vi "ExecuteMacrosRead.vi"(8 "error in (no error)":errorcluster, 11 "StepMotor in":refnum<class "StepMotor.lvclass">) -> (0 "error out":errorcluster, 2 "Значение":dbl, 3 "StepMotor out":refnum<class "StepMotor.lvclass">)   [LabVIEW 2010, in "StepMotor.lvclass"]
uses:
  StepMotor.lvclass
  StepMotor.lvclass/StepMotor.ctl
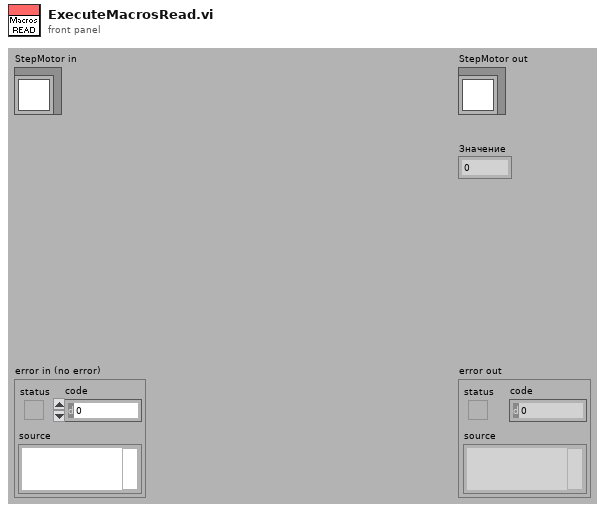
[diagram p1: front panel]
types:
  T1 = enum32{"cp1", "cp2", "cp3", "cp4", "cp5", "cp6", "cp7", "cp8", "cp9", "cp10", "cp11", "cp12", "vp1", "vp2", "vp16", "vp3", "vp4", "vp5", "vp6", "vp7", "vp8", "vp9", "vp10", "vp11", "vp12", "vp13", "vp14", "vp15", "vp17", "vp18", "vp19", "vp20", "vp21", "vp22", "vp23", "vp24", "vp25", "vp26", "pp1", "pp2", "pp3", "pp5", "pp6", "pp7", "pp8", "pp9", "pp10", "pp11", "ss1", "ss2", "ss3", "ss4", "ss5", "ss6", "ss7", "ss8", "ss9", "ss10", "ss11", "ss12", "ss13", "ss14", "ss15", "si1", "si2", "ss16", "ss17", "ss18", "ct1", "ct2", "ct3", "dd1", "dd6", "dd3", "dd9", "dd2", "dd4", "dd5", "dd21", "dd7", "dd8", "dd20", "dd10", "dd19", "dd12", "dd11", "dd13", "dd14", "dd15", "dd16", "dd17", "dd18", "dd22", "dd23", "dd24", "dd25", "dd26", "dd27", "dd28", "dd29", "dd30", "dd31", "dd32", "dd33", "dd34", "st1", "st2", "st3", "st4", "st5", "st6", "st7", "st8", "st9", "st10", "st11", "st12", "st13", "st14", "tp1", "tp3", "tp2", "tp5", "tp6", "ip0", "ip1", "ip2", "ip3", "ip4", "ip5", "ip6", "ip7", "ip8", "ip9", "ip10", "ip11", "ip12", "ip13", "ip14", "ip15", "ip16", "ip17", "ip18", "ip19", "ip20", "ep1", "ep2", "ep3", "ep4", "ep5", "ep6", "ep7", "up0", "up1", "up2", "up3", "up4", "up5", "up6", "up7", "up8", "up9", "up10", "up11", "up12", "up13", "up14", "up15", "up16", "up17", "up18", "up19", "up20", "up21", "up22", "up23", "up24", "io0", "io1", "io2", "io3", "io4", "io5", "io6", "io7", "io8", "io9", "io10", "io11", "io12", "io13", "io14", "pd1", "pd2", "pd3", "pd4", "pd5", "pd6", "pd7", "pd8", "pd9", "pd10", "pd11", "pd12", "pd13", "pd14", "pd15", "pd16", "pd17", "pd18", "pd19", " "}
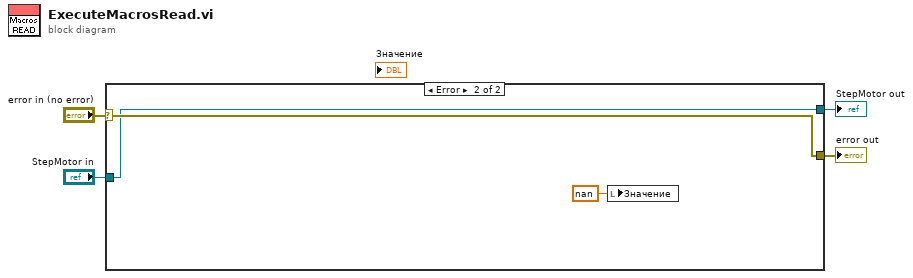
[diagram p0: block diagram]
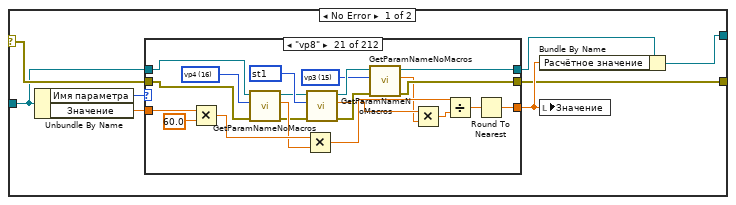
[diagram p2: hidden frame]
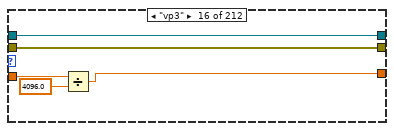
[diagram p18: hidden frame]
diagram:
  n1 = case shown="Error" "error in (no error)" {
    selector: "error in (no error)" -> [w10 w692]
    tunnel: [w9 w692] -> w3
    tunnel: [w12 w691] -> w1
    tunnel: "StepMotor in" -> [w8 w691]
    frame No Error {
      n2 = Unbundle By Name(w8) -> ("Имя параметра"=w5:T1, "Значение"=w6:dbl)
      n3 = case shown="\"vp8\"" w5 {
        tunnel: w6 -> [w15 w18 w21 w24 w27 w30 w33 w36 w39 w42 w45 w48 w51 w54 w57 w60 w63 w68 w71 w74 w83 w98 w101 w104 w107 w110 w124 w129 w132 w135 w138 w141 w144 w147 w150 w153 w156 w159 w162 w165 w168 w171 w174 w177 w180 w183 w186 w189 w192 w195 w198 w201 w204 w207 w210 w213 w216 w219 w222 w225 w228 w231 w234 w237 w240 w243 w246 w249 w252 w257 w260 w267 w270 w273 w276 w279 w282 w285 w288 w291 w294 w297 w301 w305 w308 w311 w314 w317 w320 w323 w326 w329 w332 w335 w338 w341 w344 w347 w350 w353 w356 w359 w362 w365 w368 w371 w374 w377 w380 w383 w386 w389 w392 w395 w398 w401 w404 w407 w410 w413 w416 w419 w422 w425 w428 w431 w434 w437 w440 w443 w446 w449 w452 w455 w458 w461 w464 w467 w470 w473 w476 w479 w482 w485 w488 w491 w494 w497 w500 w503 w506 w509 w512 w515 w518 w521 w524 w527 w530 w533 w536 w539 w542 w545 w548 w551 w554 w557 w560 w563 w566 w569 w572 w575 w578 w581 w584 w587 w590 w593 w596 w599 w602 w605 w608 w611 w614 w617 w620 w623 w626 w629 w632 w635 w638 w641 w644 w647 w650 w653 w656 w659 w662 w665 w668 w671 w674 w677 w680 w683 w686 w689]
        tunnel: [w15 w18 w21 w24 w27 w30 w33 w36 w39 w42 w45 w48 w51 w54 w57 w58 w63 w68 w71 w74 w84 w98 w101 w104 w107 w110 w111 w129 w132 w135 w138 w141 w144 w147 w150 w153 w156 w159 w162 w165 w168 w171 w174 w177 w180 w183 w186 w189 w192 w195 w198 w201 w204 w207 w210 w213 w216 w219 w222 w225 w228 w231 w234 w237 w240 w243 w246 w249 w252 w256 w260 w263 w270 w273 w276 w279 w282 w285 w288 w291 w294 w297 w300 w305 w308 w311 w314 w317 w320 w323 w326 w329 w332 w335 w338 w341 w344 w347 w350 w353 w356 w359 w362 w365 w368 w371 w374 w377 w380 w383 w386 w389 w392 w395 w398 w401 w404 w407 w410 w413 w416 w419 w422 w425 w428 w431 w434 w437 w440 w443 w446 w449 w452 w455 w458 w461 w464 w467 w470 w473 w476 w479 w482 w485 w488 w491 w494 w497 w500 w503 w506 w509 w512 w515 w518 w521 w524 w527 w530 w533 w536 w539 w542 w545 w548 w551 w554 w557 w560 w563 w566 w569 w572 w575 w578 w581 w584 w587 w590 w593 w596 w599 w602 w605 w608 w611 w614 w617 w620 w623 w626 w629 w632 w635 w638 w641 w644 w647 w650 w653 w656 w659 w662 w665 w668 w671 w674 w677 w680 w683 w686 w689] -> w11
        tunnel: w10 -> [w13 w16 w19 w22 w25 w28 w31 w34 w37 w40 w43 w46 w49 w52 w55 w61 w64 w66 w69 w72 w86 w96 w99 w102 w105 w108 w117 w127 w130 w133 w136 w139 w142 w145 w148 w151 w154 w157 w160 w163 w166 w169 w172 w175 w178 w181 w184 w187 w190 w193 w196 w199 w202 w205 w208 w211 w214 w217 w220 w223 w226 w229 w232 w235 w238 w241 w244 w247 w250 w253 w258 w261 w268 w271 w274 w277 w280 w283 w286 w289 w292 w295 w298 w303 w306 w309 w312 w315 w318 w321 w324 w327 w330 w333 w336 w339 w342 w345 w348 w351 w354 w357 w360 w363 w366 w369 w372 w375 w378 w381 w384 w387 w390 w393 w396 w399 w402 w405 w408 w411 w414 w417 w420 w423 w426 w429 w432 w435 w438 w441 w444 w447 w450 w453 w456 w459 w462 w465 w468 w471 w474 w477 w480 w483 w486 w489 w492 w495 w498 w501 w504 w507 w510 w513 w516 w519 w522 w525 w528 w531 w534 w537 w540 w543 w546 w549 w552 w555 w558 w561 w564 w567 w570 w573 w576 w579 w582 w585 w588 w591 w594 w597 w600 w603 w606 w609 w612 w615 w618 w621 w624 w627 w630 w633 w636 w639 w642 w645 w648 w651 w654 w657 w660 w663 w666 w669 w672 w675 w678 w681 w684 w687]
        tunnel: [w13 w16 w19 w22 w25 w28 w31 w34 w37 w40 w43 w46 w49 w52 w55 w61 w64 w66 w69 w72 w78 w96 w99 w102 w105 w108 w115 w127 w130 w133 w136 w139 w142 w145 w148 w151 w154 w157 w160 w163 w166 w169 w172 w175 w178 w181 w184 w187 w190 w193 w196 w199 w202 w205 w208 w211 w214 w217 w220 w223 w226 w229 w232 w235 w238 w241 w244 w247 w250 w253 w258 w261 w268 w271 w274 w277 w280 w283 w286 w289 w292 w295 w298 w303 w306 w309 w312 w315 w318 w321 w324 w327 w330 w333 w336 w339 w342 w345 w348 w351 w354 w357 w360 w363 w366 w369 w372 w375 w378 w381 w384 w387 w390 w393 w396 w399 w402 w405 w408 w411 w414 w417 w420 w423 w426 w429 w432 w435 w438 w441 w444 w447 w450 w453 w456 w459 w462 w465 w468 w471 w474 w477 w480 w483 w486 w489 w492 w495 w498 w501 w504 w507 w510 w513 w516 w519 w522 w525 w528 w531 w534 w537 w540 w543 w546 w549 w552 w555 w558 w561 w564 w567 w570 w573 w576 w579 w582 w585 w588 w591 w594 w597 w600 w603 w606 w609 w612 w615 w618 w621 w624 w627 w630 w633 w636 w639 w642 w645 w648 w651 w654 w657 w660 w663 w666 w669 w672 w675 w678 w681 w684 w687] -> w9
        tunnel: w8 -> [w14 w17 w20 w23 w26 w29 w32 w35 w38 w41 w44 w47 w50 w53 w56 w62 w65 w67 w70 w73 w85 w97 w100 w103 w106 w109 w114 w128 w131 w134 w137 w140 w143 w146 w149 w152 w155 w158 w161 w164 w167 w170 w173 w176 w179 w182 w185 w188 w191 w194 w197 w200 w203 w206 w209 w212 w215 w218 w221 w224 w227 w230 w233 w236 w239 w242 w245 w248 w251 w254 w259 w262 w269 w272 w275 w278 w281 w284 w287 w290 w293 w296 w299 w304 w307 w310 w313 w316 w319 w322 w325 w328 w331 w334 w337 w340 w343 w346 w349 w352 w355 w358 w361 w364 w367 w370 w373 w376 w379 w382 w385 w388 w391 w394 w397 w400 w403 w406 w409 w412 w415 w418 w421 w424 w427 w430 w433 w436 w439 w442 w445 w448 w451 w454 w457 w460 w463 w466 w469 w472 w475 w478 w481 w484 w487 w490 w493 w496 w499 w502 w505 w508 w511 w514 w517 w520 w523 w526 w529 w532 w535 w538 w541 w544 w547 w550 w553 w556 w559 w562 w565 w568 w571 w574 w577 w580 w583 w586 w589 w592 w595 w598 w601 w604 w607 w610 w613 w616 w619 w622 w625 w628 w631 w634 w637 w640 w643 w646 w649 w652 w655 w658 w661 w664 w667 w670 w673 w676 w679 w682 w685 w688]
        tunnel: [w14 w17 w20 w23 w26 w29 w32 w35 w38 w41 w44 w47 w50 w53 w56 w62 w65 w67 w70 w73 w79 w97 w100 w103 w106 w109 w113 w128 w131 w134 w137 w140 w143 w146 w149 w152 w155 w158 w161 w164 w167 w170 w173 w176 w179 w182 w185 w188 w191 w194 w197 w200 w203 w206 w209 w212 w215 w218 w221 w224 w227 w230 w233 w236 w239 w242 w245 w248 w251 w254 w259 w262 w269 w272 w275 w278 w281 w284 w287 w290 w293 w296 w299 w304 w307 w310 w313 w316 w319 w322 w325 w328 w331 w334 w337 w340 w343 w346 w349 w352 w355 w358 w361 w364 w367 w370 w373 w376 w379 w382 w385 w388 w391 w394 w397 w400 w403 w406 w409 w412 w415 w418 w421 w424 w427 w430 w433 w436 w439 w442 w445 w448 w451 w454 w457 w460 w463 w466 w469 w472 w475 w478 w481 w484 w487 w490 w493 w496 w499 w502 w505 w508 w511 w514 w517 w520 w523 w526 w529 w532 w535 w538 w541 w544 w547 w550 w553 w556 w559 w562 w565 w568 w571 w574 w577 w580 w583 w586 w589 w592 w595 w598 w601 w604 w607 w610 w613 w616 w619 w622 w625 w628 w631 w634 w637 w640 w643 w646 w649 w652 w655 w658 w661 w664 w667 w670 w673 w676 w679 w682 w685 w688] -> w7
        frame "cp1" {
        }
        frame "cp2" {
        }
        frame "cp3" {
        }
        frame "cp4" {
        }
        frame "cp5" {
        }
        frame "cp6" {
        }
        frame "cp7" {
        }
        frame "cp8" {
        }
        frame "cp9" {
        }
        frame "cp10" {
        }
        frame "cp11" {
        }
        frame "cp12" {
        }
        frame "vp1" {
        }
        frame "vp2" {
        }
        frame "vp16" {
        }
        frame "vp3" {
          n4 = Divide(x=w60, y=4096.0) -> (x/y=w58:dbl)
        }
        frame "vp4" {
        }
        frame "vp5" {
        }
        frame "vp6" {
        }
        frame "vp7" {
        }
        frame "vp8" {
          w80 = 15 items=["cp1", "cp2", "cp3", "cp4", "cp5", "cp6", "cp7", "cp8", "cp9", "cp10", "cp11", "cp12", "vp1", "vp2", "vp16", "vp3", "vp4", "vp5", "vp6", "vp7", "vp8", "vp9", "vp10", "vp11", "vp12", "vp13", "vp14", "vp15", "vp17", "vp18", "vp19", "vp20", "vp21", "vp22", "vp23", "vp24", "vp25", "vp26", "pp1", "pp2", "pp3", "pp5", "pp6", "pp7", "pp8", "pp9", "pp10", "pp11", "ss1", "ss2", "ss3", "ss4", "ss5", "ss6", "ss7", "ss8", "ss9", "ss10", "ss11", "ss12", "ss13", "ss14", "ss15", "si1", "si2", "ss16", "ss17", "ss18", "ct1", "ct2", "ct3", "dd1", "dd6", "dd3", "dd9", "dd2", "dd4", "dd5", "dd21", "dd7", "dd8", "dd20", "dd10", "dd19", "dd12", "dd11", "dd13", "dd14", "dd15", "dd16", "dd17", "dd18", "dd22", "dd23", "dd24", "dd25", "dd26", "dd27", "dd28", "dd29", "dd30", "dd31", "dd32", "dd33", "dd34", "st1", "st2", "st3", "st4", "st5", "st6", "st7", "st8", "st9", "st10", "st11", "st12", "st13", "st14", "tp1", "tp3", "tp2", "tp5", "tp6", "ip0", "ip1", "ip2", "ip3", "ip4", "ip5", "ip6", "ip7", "ip8", "ip9", "ip10", "ip11", "ip12", "ip13", "ip14", "ip15", "ip16", "ip17", "ip18", "ip19", "ip20", "ep1", "ep2", "ep3", "ep4", "ep5", "ep6", "ep7", "up0", "up1", "up2", "up3", "up4", "up5", "up6", "up7", "up8", "up9", "up10", "up11", "up12", "up13", "up14", "up15", "up16", "up17", "up18", "up19", "up20", "up21", "up22", "up23", "up24", "io0", "io1", "io2", "io3", "io4", "io5", "io6", "io7", "io8", "io9", "io10", "io11", "io12", "io13", "io14", "pd1", "pd2", "pd3", "pd4", "pd5", "pd6", "pd7", "pd8", "pd9", "pd10", "pd11", "pd12", "pd13", "pd14", "pd15", "pd16", "pd17", "pd18", "pd19"] ("Имя параметра")
          w94 = 16 items=["cp1", "cp2", "cp3", "cp4", "cp5", "cp6", "cp7", "cp8", "cp9", "cp10", "cp11", "cp12", "vp1", "vp2", "vp16", "vp3", "vp4", "vp5", "vp6", "vp7", "vp8", "vp9", "vp10", "vp11", "vp12", "vp13", "vp14", "vp15", "vp17", "vp18", "vp19", "vp20", "vp21", "vp22", "vp23", "vp24", "vp25", "vp26", "pp1", "pp2", "pp3", "pp5", "pp6", "pp7", "pp8", "pp9", "pp10", "pp11", "ss1", "ss2", "ss3", "ss4", "ss5", "ss6", "ss7", "ss8", "ss9", "ss10", "ss11", "ss12", "ss13", "ss14", "ss15", "si1", "si2", "ss16", "ss17", "ss18", "ct1", "ct2", "ct3", "dd1", "dd6", "dd3", "dd9", "dd2", "dd4", "dd5", "dd21", "dd7", "dd8", "dd20", "dd10", "dd19", "dd12", "dd11", "dd13", "dd14", "dd15", "dd16", "dd17", "dd18", "dd22", "dd23", "dd24", "dd25", "dd26", "dd27", "dd28", "dd29", "dd30", "dd31", "dd32", "dd33", "dd34", "st1", "st2", "st3", "st4", "st5", "st6", "st7", "st8", "st9", "st10", "st11", "st12", "st13", "st14", "tp1", "tp3", "tp2", "tp5", "tp6", "ip0", "ip1", "ip2", "ip3", "ip4", "ip5", "ip6", "ip7", "ip8", "ip9", "ip10", "ip11", "ip12", "ip13", "ip14", "ip15", "ip16", "ip17", "ip18", "ip19", "ip20", "ep1", "ep2", "ep3", "ep4", "ep5", "ep6", "ep7", "up0", "up1", "up2", "up3", "up4", "up5", "up6", "up7", "up8", "up9", "up10", "up11", "up12", "up13", "up14", "up15", "up16", "up17", "up18", "up19", "up20", "up21", "up22", "up23", "up24", "io0", "io1", "io2", "io3", "io4", "io5", "io6", "io7", "io8", "io9", "io10", "io11", "io12", "io13", "io14", "pd1", "pd2", "pd3", "pd4", "pd5", "pd6", "pd7", "pd8", "pd9", "pd10", "pd11", "pd12", "pd13", "pd14", "pd15", "pd16", "pd17", "pd18", "pd19"] ("Имя параметра")
          w95 = 105 items=["cp1", "cp2", "cp3", "cp4", "cp5", "cp6", "cp7", "cp8", "cp9", "cp10", "cp11", "cp12", "vp1", "vp2", "vp16", "vp3", "vp4", "vp5", "vp6", "vp7", "vp8", "vp9", "vp10", "vp11", "vp12", "vp13", "vp14", "vp15", "vp17", "vp18", "vp19", "vp20", "vp21", "vp22", "vp23", "vp24", "vp25", "vp26", "pp1", "pp2", "pp3", "pp5", "pp6", "pp7", "pp8", "pp9", "pp10", "pp11", "ss1", "ss2", "ss3", "ss4", "ss5", "ss6", "ss7", "ss8", "ss9", "ss10", "ss11", "ss12", "ss13", "ss14", "ss15", "si1", "si2", "ss16", "ss17", "ss18", "ct1", "ct2", "ct3", "dd1", "dd6", "dd3", "dd9", "dd2", "dd4", "dd5", "dd21", "dd7", "dd8", "dd20", "dd10", "dd19", "dd12", "dd11", "dd13", "dd14", "dd15", "dd16", "dd17", "dd18", "dd22", "dd23", "dd24", "dd25", "dd26", "dd27", "dd28", "dd29", "dd30", "dd31", "dd32", "dd33", "dd34", "st1", "st2", "st3", "st4", "st5", "st6", "st7", "st8", "st9", "st10", "st11", "st12", "st13", "st14", "tp1", "tp3", "tp2", "tp5", "tp6", "ip0", "ip1", "ip2", "ip3", "ip4", "ip5", "ip6", "ip7", "ip8", "ip9", "ip10", "ip11", "ip12", "ip13", "ip14", "ip15", "ip16", "ip17", "ip18", "ip19", "ip20", "ep1", "ep2", "ep3", "ep4", "ep5", "ep6", "ep7", "up0", "up1", "up2", "up3", "up4", "up5", "up6", "up7", "up8", "up9", "up10", "up11", "up12", "up13", "up14", "up15", "up16", "up17", "up18", "up19", "up20", "up21", "up22", "up23", "up24", "io0", "io1", "io2", "io3", "io4", "io5", "io6", "io7", "io8", "io9", "io10", "io11", "io12", "io13", "io14", "pd1", "pd2", "pd3", "pd4", "pd5", "pd6", "pd7", "pd8", "pd9", "pd10", "pd11", "pd12", "pd13", "pd14", "pd15", "pd16", "pd17", "pd18", "pd19"] ("Имя параметра")
          n5 = Multiply(x=w83, y=60.0) -> (x*y=w92:dbl)
          n6 = call-dynamic "GetParamNameNoMacros.vi"("error in (no error)"=w86, "Имя параметра"=w94, "StepMotor in"=w85) -> ("error out"=w88:errorcluster, "Значение"=w91:dbl, "StepMotor out"=w89:refnum<class "StepMotor.lvclass">)  [unwired: 6 in]
          n7 = Multiply(x=w92, y=w91) -> (x*y=w90:dbl)
          n8 = call-dynamic "GetParamNameNoMacros.vi"("error in (no error)"=w88, "Имя параметра"=w95, "StepMotor in"=w89) -> ("error out"=w81:errorcluster, "Значение"=w77:dbl, "StepMotor out"=w82:refnum<class "StepMotor.lvclass">)  [unwired: 6 in]
          n9 = call-dynamic "GetParamNameNoMacros.vi"("error in (no error)"=w81, "Имя параметра"=w80, "StepMotor in"=w82) -> ("error out"=w78:errorcluster, "Значение"=w75:dbl, "StepMotor out"=w79:refnum<class "StepMotor.lvclass">)  [unwired: 6 in]
          n10 = Multiply(x=w77, y=w75) -> (x*y=w76:dbl)
          n11 = Divide(x=w90, y=w76) -> (x/y=w87:dbl)
          n12 = Round To Nearest(number=w87) -> (nearest integer value=w84:dbl)
        }
        frame "vp9" {
        }
        frame "vp10" {
        }
        frame "vp11" {
        }
        frame "vp12" {
        }
        frame "vp13" {
        }
        frame "vp14" {
          w125 = 16 items=["cp1", "cp2", "cp3", "cp4", "cp5", "cp6", "cp7", "cp8", "cp9", "cp10", "cp11", "cp12", "vp1", "vp2", "vp16", "vp3", "vp4", "vp5", "vp6", "vp7", "vp8", "vp9", "vp10", "vp11", "vp12", "vp13", "vp14", "vp15", "vp17", "vp18", "vp19", "vp20", "vp21", "vp22", "vp23", "vp24", "vp25", "vp26", "pp1", "pp2", "pp3", "pp5", "pp6", "pp7", "pp8", "pp9", "pp10", "pp11", "ss1", "ss2", "ss3", "ss4", "ss5", "ss6", "ss7", "ss8", "ss9", "ss10", "ss11", "ss12", "ss13", "ss14", "ss15", "si1", "si2", "ss16", "ss17", "ss18", "ct1", "ct2", "ct3", "dd1", "dd6", "dd3", "dd9", "dd2", "dd4", "dd5", "dd21", "dd7", "dd8", "dd20", "dd10", "dd19", "dd12", "dd11", "dd13", "dd14", "dd15", "dd16", "dd17", "dd18", "dd22", "dd23", "dd24", "dd25", "dd26", "dd27", "dd28", "dd29", "dd30", "dd31", "dd32", "dd33", "dd34", "st1", "st2", "st3", "st4", "st5", "st6", "st7", "st8", "st9", "st10", "st11", "st12", "st13", "st14", "tp1", "tp3", "tp2", "tp5", "tp6", "ip0", "ip1", "ip2", "ip3", "ip4", "ip5", "ip6", "ip7", "ip8", "ip9", "ip10", "ip11", "ip12", "ip13", "ip14", "ip15", "ip16", "ip17", "ip18", "ip19", "ip20", "ep1", "ep2", "ep3", "ep4", "ep5", "ep6", "ep7", "up0", "up1", "up2", "up3", "up4", "up5", "up6", "up7", "up8", "up9", "up10", "up11", "up12", "up13", "up14", "up15", "up16", "up17", "up18", "up19", "up20", "up21", "up22", "up23", "up24", "io0", "io1", "io2", "io3", "io4", "io5", "io6", "io7", "io8", "io9", "io10", "io11", "io12", "io13", "io14", "pd1", "pd2", "pd3", "pd4", "pd5", "pd6", "pd7", "pd8", "pd9", "pd10", "pd11", "pd12", "pd13", "pd14", "pd15", "pd16", "pd17", "pd18", "pd19"] ("Имя параметра")
          w126 = 105 items=["cp1", "cp2", "cp3", "cp4", "cp5", "cp6", "cp7", "cp8", "cp9", "cp10", "cp11", "cp12", "vp1", "vp2", "vp16", "vp3", "vp4", "vp5", "vp6", "vp7", "vp8", "vp9", "vp10", "vp11", "vp12", "vp13", "vp14", "vp15", "vp17", "vp18", "vp19", "vp20", "vp21", "vp22", "vp23", "vp24", "vp25", "vp26", "pp1", "pp2", "pp3", "pp5", "pp6", "pp7", "pp8", "pp9", "pp10", "pp11", "ss1", "ss2", "ss3", "ss4", "ss5", "ss6", "ss7", "ss8", "ss9", "ss10", "ss11", "ss12", "ss13", "ss14", "ss15", "si1", "si2", "ss16", "ss17", "ss18", "ct1", "ct2", "ct3", "dd1", "dd6", "dd3", "dd9", "dd2", "dd4", "dd5", "dd21", "dd7", "dd8", "dd20", "dd10", "dd19", "dd12", "dd11", "dd13", "dd14", "dd15", "dd16", "dd17", "dd18", "dd22", "dd23", "dd24", "dd25", "dd26", "dd27", "dd28", "dd29", "dd30", "dd31", "dd32", "dd33", "dd34", "st1", "st2", "st3", "st4", "st5", "st6", "st7", "st8", "st9", "st10", "st11", "st12", "st13", "st14", "tp1", "tp3", "tp2", "tp5", "tp6", "ip0", "ip1", "ip2", "ip3", "ip4", "ip5", "ip6", "ip7", "ip8", "ip9", "ip10", "ip11", "ip12", "ip13", "ip14", "ip15", "ip16", "ip17", "ip18", "ip19", "ip20", "ep1", "ep2", "ep3", "ep4", "ep5", "ep6", "ep7", "up0", "up1", "up2", "up3", "up4", "up5", "up6", "up7", "up8", "up9", "up10", "up11", "up12", "up13", "up14", "up15", "up16", "up17", "up18", "up19", "up20", "up21", "up22", "up23", "up24", "io0", "io1", "io2", "io3", "io4", "io5", "io6", "io7", "io8", "io9", "io10", "io11", "io12", "io13", "io14", "pd1", "pd2", "pd3", "pd4", "pd5", "pd6", "pd7", "pd8", "pd9", "pd10", "pd11", "pd12", "pd13", "pd14", "pd15", "pd16", "pd17", "pd18", "pd19"] ("Имя параметра")
          n13 = Multiply(x=w124, y=60.0) -> (x*y=w122:dbl)
          n14 = call-dynamic "GetParamNameNoMacros.vi"("error in (no error)"=w117, "Имя параметра"=w125, "StepMotor in"=w114) -> ("error out"=w116:errorcluster, "Значение"=w121:dbl, "StepMotor out"=w118:refnum<class "StepMotor.lvclass">)  [unwired: 6 in]
          n15 = Multiply(x=w122, y=w121) -> (x*y=w120:dbl)
          n16 = call-dynamic "GetParamNameNoMacros.vi"("error in (no error)"=w116, "Имя параметра"=w126, "StepMotor in"=w118) -> ("error out"=w115:errorcluster, "Значение"=w119:dbl, "StepMotor out"=w113:refnum<class "StepMotor.lvclass">)  [unwired: 6 in]
          n17 = Divide(x=w120, y=w119) -> (x/y=w112:dbl)
          n18 = Round To Nearest(number=w112) -> (nearest integer value=w111:dbl)
        }
        frame "vp15" {
        }
        frame "vp17" {
        }
        frame "vp18" {
        }
        frame "vp19" {
        }
        frame "vp20" {
        }
        frame "vp21" {
        }
        frame "vp22" {
        }
        frame "vp23" {
        }
        frame "vp24" {
        }
        frame "vp25" {
        }
        frame "vp26" {
        }
        frame "pp1" {
        }
        frame "pp2" {
        }
        frame "pp3" {
        }
        frame "pp5" {
        }
        frame "pp6" {
        }
        frame "pp7" {
        }
        frame "pp8" {
        }
        frame "pp9" {
        }
        frame "pp10" {
        }
        frame "pp11" {
        }
        frame "ss1" {
        }
        frame "ss2" {
        }
        frame "ss3" {
        }
        frame "ss4" {
        }
        frame "ss5" {
        }
        frame "ss6" {
        }
        frame "ss7" {
        }
        frame "ss8" {
        }
        frame "ss9" {
        }
        frame "ss10" {
        }
        frame "ss11" {
        }
        frame "ss12" {
        }
        frame "ss13" {
        }
        frame "ss14" {
        }
        frame "ss15" {
        }
        frame "si1" {
        }
        frame "si2" {
        }
        frame "ss16" {
        }
        frame "ss17" {
        }
        frame "ss18" {
        }
        frame "ct1" {
        }
        frame "ct2" {
          n19 = Divide(x=w257, y=4096.0) -> (x/y=w256:dbl)
        }
        frame "ct3" {
        }
        frame "dd1" {
          n20 = Multiply(x=w267, y=u32 5) -> (x*y=w265:dbl)
          n21 = Divide(x=w265, y=u32 2047) -> (x/y=w263:dbl)
        }
        frame "dd6" {
        }
        frame "dd3" {
        }
        frame "dd9" {
        }
        frame "dd2" {
        }
        frame "dd4" {
        }
        frame "dd5" {
        }
        frame "dd21" {
        }
        frame "dd7" {
        }
        frame "dd8" {
        }
        frame "dd20" {
        }
        frame "dd10" {
          n22 = Divide(x=w301, y=u32 128) -> (x/y=w300:dbl)
        }
        frame "dd19" {
        }
        frame "dd12" {
        }
        frame "dd11" {
        }
        frame "dd13" {
        }
        frame "dd14" {
        }
        frame "dd15" {
        }
        frame "dd16" {
        }
        frame "dd17" {
        }
        frame "dd18" {
        }
        frame "dd22" {
        }
        frame "dd23" {
        }
        frame "dd24" {
        }
        frame "dd25" {
        }
        frame "dd26" {
        }
        frame "dd27" {
        }
        frame "dd28" {
        }
        frame "dd29" {
        }
        frame "dd30" {
        }
        frame "dd31" {
        }
        frame "dd32" {
        }
        frame "dd33" {
        }
        frame "dd34" {
        }
        frame "st1" {
        }
        frame "st2" {
        }
        frame "st3" {
        }
        frame "st4" {
        }
        frame "st5" {
        }
        frame "st6" {
        }
        frame "st7" {
        }
        frame "st8" {
        }
        frame "st9" {
        }
        frame "st10" {
        }
        frame "st11" {
        }
        frame "st12" {
        }
        frame "st13" {
        }
        frame "st14" {
        }
        frame "tp1" {
        }
        frame "tp3" {
        }
        frame "tp2" {
        }
        frame "tp5" {
        }
        frame "tp6" {
        }
        frame "ip0" {
        }
        frame "ip1" {
        }
        frame "ip2" {
        }
        frame "ip3" {
        }
        frame "ip4" {
        }
        frame "ip5" {
        }
        frame "ip6" {
        }
        frame "ip7" {
        }
        frame "ip8" {
        }
        frame "ip9" {
        }
        frame "ip10" {
        }
        frame "ip11" {
        }
        frame "ip12" {
        }
        frame "ip13" {
        }
        frame "ip14" {
        }
        frame "ip15" {
        }
        frame "ip16" {
        }
        frame "ip17" {
        }
        frame "ip18" {
        }
        frame "ip19" {
        }
        frame "ip20" {
        }
        frame "ep1" {
        }
        frame "ep2" {
        }
        frame "ep3" {
        }
        frame "ep4" {
        }
        frame "ep5" {
        }
        frame "ep6" {
        }
        frame "ep7" {
        }
        frame "up0" {
        }
        frame "up1" {
        }
        frame "up2" {
        }
        frame "up3" {
        }
        frame "up4" {
        }
        frame "up5" {
        }
        frame "up6" {
        }
        frame "up7" {
        }
        frame "up8" {
        }
        frame "up9" {
        }
        frame "up10" {
        }
        frame "up11" {
        }
        frame "up12" {
        }
        frame "up13" {
        }
        frame "up14" {
        }
        frame "up15" {
        }
        frame "up16" {
        }
        frame "up17" {
        }
        frame "up18" {
        }
        frame "up19" {
        }
        frame "up20" {
        }
        frame "up21" {
        }
        frame "up22" {
        }
        frame "up23" {
        }
        frame "up24" {
        }
        frame "io0" {
        }
        frame "io1" {
        }
        frame "io2" {
        }
        frame "io3" {
        }
        frame "io4" {
        }
        frame "io5" {
        }
        frame "io6" {
        }
        frame "io7" {
        }
        frame "io8" {
        }
        frame "io9" {
        }
        frame "io10" {
        }
        frame "io11" {
        }
        frame "io12" {
        }
        frame "io13" {
        }
        frame "io14" {
        }
        frame "pd1" {
        }
        frame "pd2" {
        }
        frame "pd3" {
        }
        frame "pd4" {
        }
        frame "pd5" {
        }
        frame "pd6" {
        }
        frame "pd7" {
        }
        frame "pd8" {
        }
        frame "pd9" {
        }
        frame "pd10" {
        }
        frame "pd11" {
        }
        frame "pd12" {
        }
        frame "pd13" {
        }
        frame "pd14" {
        }
        frame "pd15" {
        }
        frame "pd16" {
        }
        frame "pd17" {
        }
        frame "pd18" {
        }
        frame "pd19" {
        }
        frame " ", Default {
        }
      }
      n23 = Bundle By Name(cluster=w7, "Расчётное значение"=w11) -> (w12:refnum<class "StepMotor.lvclass">)
      n24 = local write "Значение"(w11) -> ()
    }
    frame Error {
      n25 = local write "Значение"(nan ("Значение")) -> ()
    }
  }
  "error out" <- w3
  "StepMotor out" <- w1
